vi "PCO_GetCameraDescription.vi"(8 "error in (no error)":errorcluster {"code" format="%x"}, 11 "ph":u64) -> (0 "error out":errorcluster {"code" format="%x"}, 1 "strDescription":T1 {"wSensorTypeDESC" format="%x"; "wSensorSubTypeDESC" format="%x"; "wColorPatternDESC" format="%x"; "wPatternTypeDESC" format="%x"; "dwGeneralCapsDESC1" format="%x"; "dwGeneralCapsDESC2" format="%x"; "dwGeneralCapsDESC3" format="%x"; "dwGeneralCapsDESC4" format="%x"}, 2 "ErrorMessage":i32 format="%x", 3 "ph out":u64)   [LabVIEW 2019, in "SDK.lvlib" / "CameraDescription.lvlib"]
doc: "<b>Description:</b>\nSensor and camera specific description is queried. In the returned PCO_Description structure margins for all sensor related settings and bitfields for available options of the camera are given.\n\n<b>Supported camera type:</b>\nAll cameras\n\n<b>Descriptor dependency:</b>\nNone"
uses:
  CameraDescription.lvlib
  Structures/Structures.lvlib
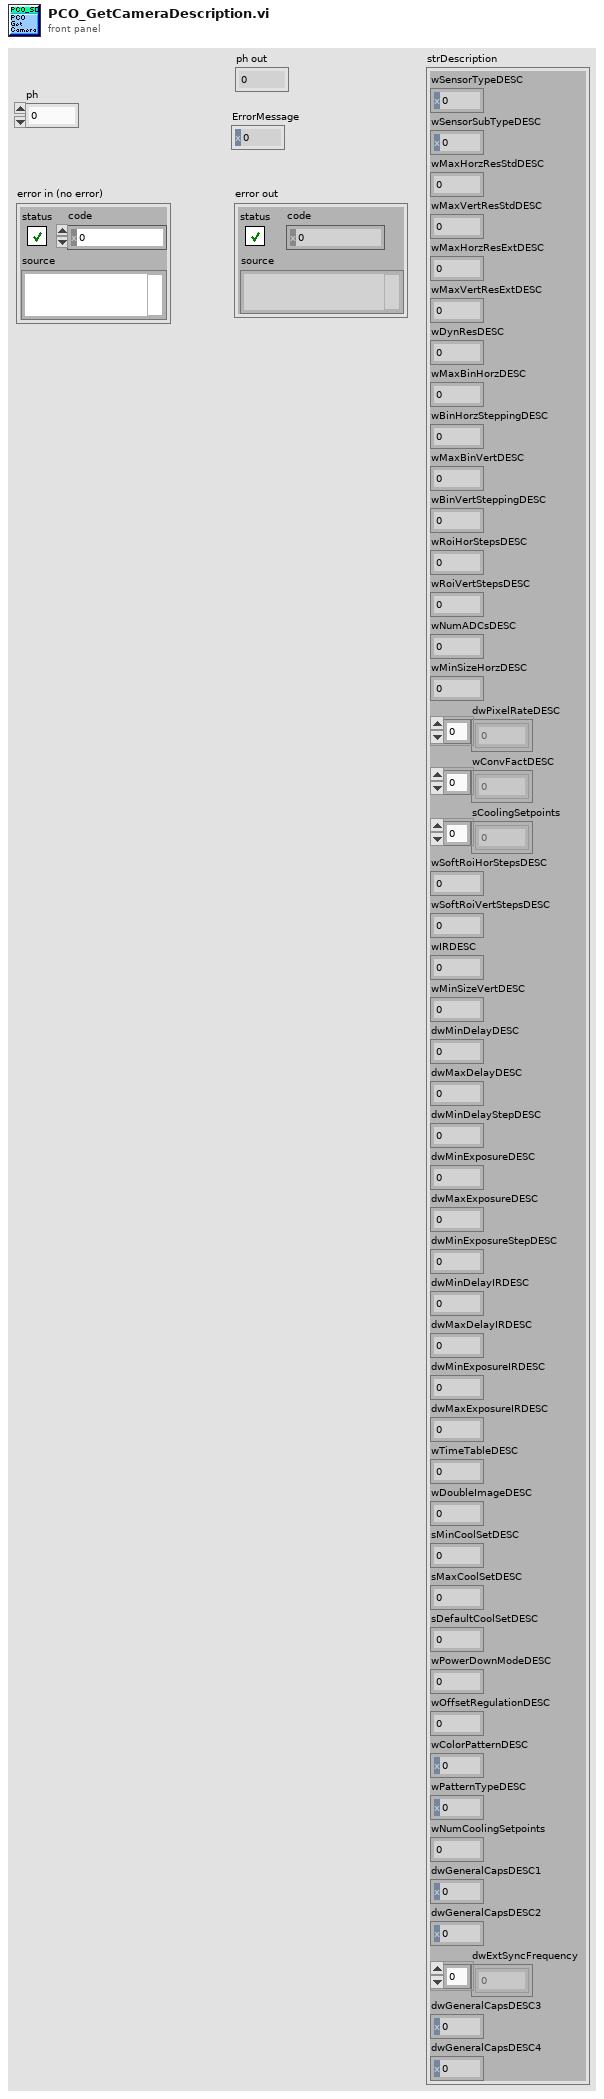
[diagram p1: front panel]
types:
  T1 = cluster{"wSensorTypeDESC":u16, "wSensorSubTypeDESC":u16, "wMaxHorzResStdDESC":u16, "wMaxVertResStdDESC":u16, "wMaxHorzResExtDESC":u16, "wMaxVertResExtDESC":u16, "wDynResDESC":u16, "wMaxBinHorzDESC":u16, "wBinHorzSteppingDESC":u16, "wMaxBinVertDESC":u16, "wBinVertSteppingDESC":u16, "wRoiHorStepsDESC":u16, "wRoiVertStepsDESC":u16, "wNumADCsDESC":u16, "wMinSizeHorzDESC":u16, "dwPixelRateDESC":u32[], "wConvFactDESC":u16[], "sCoolingSetpoints":i16[], "wSoftRoiHorStepsDESC":u16, "wSoftRoiVertStepsDESC":u16, "wIRDESC":u16, "wMinSizeVertDESC":u16, "dwMinDelayDESC":u32, "dwMaxDelayDESC":u32, "dwMinDelayStepDESC":u32, "dwMinExposureDESC":u32, "dwMaxExposureDESC":u32, "dwMinExposureStepDESC":u32, "dwMinDelayIRDESC":u32, "dwMaxDelayIRDESC":u32, "dwMinExposureIRDESC":u32, "dwMaxExposureIRDESC":u32, "wTimeTableDESC":u16, "wDoubleImageDESC":u16, "sMinCoolSetDESC":i16, "sMaxCoolSetDESC":i16, "sDefaultCoolSetDESC":i16, "wPowerDownModeDESC":u16, "wOffsetRegulationDESC":u16, "wColorPatternDESC":u16, "wPatternTypeDESC":u16, "wNumCoolingSetpoints":u16, "dwGeneralCapsDESC1":u32, "dwGeneralCapsDESC2":u32, "dwExtSyncFrequency":u32[], "dwGeneralCapsDESC3":u32, "dwGeneralCapsDESC4":u32}
  T2 = cluster{"wSize":u16, "wSensorTypeDESC":u16, "wSensorSubTypeDESC":u16, "wMaxHorzResStdDESC":u16, "wMaxVertResStdDESC":u16, "wMaxHorzResExtDESC":u16, "wMaxVertResExtDESC":u16, "wDynResDESC":u16, "wMaxBinHorzDESC":u16, "wBinHorzSteppingDESC":u16, "wMaxBinVertDESC":u16, "wBinVertSteppingDESC":u16, "wRoiHorStepsDESC":u16, "wRoiVertStepsDESC":u16, "wNumADCsDESC":u16, "wMinSizeHorzDESC":u16, "dwPixelRateDESC":cluster{u32, u32, u32, u32}, "ZZdwDummypr":cluster{u32, u32, u32, u32, u32, u32, u32, u32, u32, u32, u32, u32, u32, u32, u32, u32, u32, u32, u32, u32}, "wConvFactDESC":cluster{u16, u16, u16, u16}, "sCoolingSetpoints":cluster{i16, i16, i16, i16, i16, i16, i16, i16, i16, i16}, "ZZdwDummycv":cluster{u16, u16, u16, u16, u16, u16, u16, u16}, "wSoftRoiHorStepsDESC":u16, "wSoftRoiVertStepsDESC":u16, "wIRDESC":u16, "wMinSizeVertDESC":u16, "dwMinDelayDESC":u32, "dwMaxDelayDESC":u32, "dwMinDelayStepDESC":u32, "dwMinExposureDESC":u32, "dwMaxExposureDESC":u32, "dwMinExposureStepDESC":u32, "dwMinDelayIRDESC":u32, "dwMaxDelayIRDESC":u32, "dwMinExposureIRDESC":u32, "dwMaxExposureIRDESC":u32, "wTimeTableDESC":u16, "wDoubleImageDESC":u16, "sMinCoolSetDESC":i16, "sMaxCoolSetDESC":i16, "sDefaultCoolSetDESC":i16, "wPowerDownModeDESC":u16, "wOffsetRegulationDESC":u16, "wColorPatternDESC":u16, "wPatternTypeDESC":u16, "wDummy1":u16, "wDummy2":u16, "wNumCoolingSetpoints":u16, "dwGeneralCapsDESC1":u32, "dwGeneralCapsDESC2":u32, "dwExtSyncFrequency":cluster{u32, u32, u32, u32}, "dwGeneralCapsDESC3":u32, "dwGeneralCapsDESC4":u32, "ZZdwDummy":cluster{u32, u32, u32, u32, u32, u32, u32, u32, u32, u32, u32, u32, u32, u32, u32, u32, u32, u32, u32, u32, u32, u32, u32, u32, u32, u32, u32, u32, u32, u32, u32, u32, u32, u32, u32, u32, u32, u32, u32, u32}}
  T3 = cluster{i16, i16, i16, i16, i16, i16, i16, i16, i16, i16}
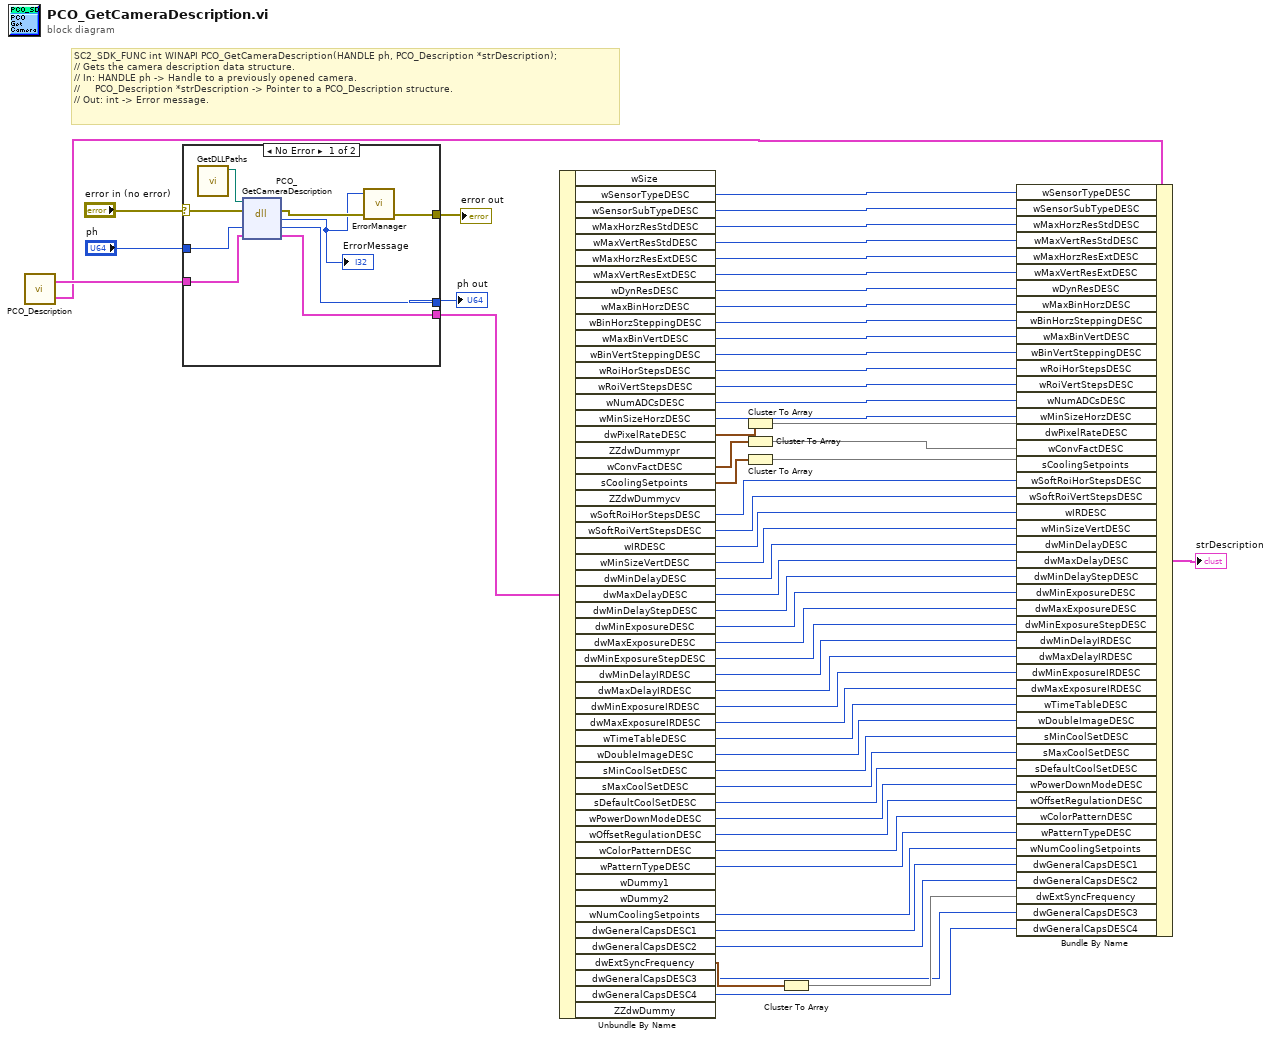
[diagram p0: block diagram]
diagram:
  # "SC2_SDK_FUNC int WINAPI PCO_GetCameraDescription(HANDLE ph, PCO_Description *strDescription);\n// Gets the camera description data structure.\n// In: HANDLE ph -> Handle to a previously opened camera.\n//     PCO_Description *strDescription -> Pointer to a PCO_Description structure.\n// Out: int -> Error message."
  n1 = call "PCO_Description.vi"() -> ("PCO_Description"=w53:T1, "PCO_Description_Raw"=w55:T2)  [unwired: 4 in, 2 out]
  n2 = case shown="No Error" "error in (no error)" {
    selector: "error in (no error)" -> [w61 w71]
    tunnel: "ph" -> [w68 w70]
    tunnel: [w67 w70] -> w58
    tunnel: w55 -> [w66 w69]
    tunnel: [w65 w69] -> w54
    tunnel: [w63 w71] -> w57
    frame No Error {
      n3 = call "GetDLLPaths.vi"() -> ("SC2_Cam_Path"=w60:path)  [unwired: 8 in, 3 out]
      n4 = dll-call lib="?" fn="PCO_GetCameraDescription"(path in=w60, error in=w61, "ph"=w68, "strDescription"=w66) -> (error out=w64:errorcluster, "return type"=w62:i32, "ph"=w67:u64, "strDescription"=w65:T2)  [unwired: 1 in, 1 out]
      "ErrorMessage" <- w62
      n5 = call "ErrorManager.vi"("error in (no error)"=w64, "error code"=w62) -> ("error out"=w63:errorcluster)  [unwired: 2 in, 1 out]
    }
    frame Error {
    }
  }
  "ph out" <- w58
  "error out" <- w57
  n6 = Unbundle By Name(w54) -> ("wSensorTypeDESC"=w51:u16, "wSensorSubTypeDESC"=w50:u16, "wMaxHorzResStdDESC"=w49:u16, "wMaxVertResStdDESC"=w48:u16, "wMaxHorzResExtDESC"=w47:u16, "wMaxVertResExtDESC"=w46:u16, "wDynResDESC"=w45:u16, "wMaxBinHorzDESC"=w44:u16, "wBinHorzSteppingDESC"=w43:u16, "wMaxBinVertDESC"=w42:u16, "wBinVertSteppingDESC"=w41:u16, "wRoiHorStepsDESC"=w40:u16, "wRoiVertStepsDESC"=w39:u16, "wNumADCsDESC"=w38:u16, "wMinSizeHorzDESC"=w37:u16, "dwPixelRateDESC"=w36:cluster{u32, u32, u32, u32}, "wConvFactDESC"=w34:cluster{u16, u16, u16, u16}, "sCoolingSetpoints"=w32:T3, "wSoftRoiHorStepsDESC"=w30:u16, "wSoftRoiVertStepsDESC"=w29:u16, "wIRDESC"=w28:u16, "wMinSizeVertDESC"=w27:u16, "dwMinDelayDESC"=w26:u32, "dwMaxDelayDESC"=w25:u32, "dwMinDelayStepDESC"=w24:u32, "dwMinExposureDESC"=w23:u32, "dwMaxExposureDESC"=w22:u32, "dwMinExposureStepDESC"=w21:u32, "dwMinDelayIRDESC"=w20:u32, "dwMaxDelayIRDESC"=w19:u32, "dwMinExposureIRDESC"=w18:u32, "dwMaxExposureIRDESC"=w17:u32, "wTimeTableDESC"=w16:u16, "wDoubleImageDESC"=w15:u16, "sMinCoolSetDESC"=w14:i16, "sMaxCoolSetDESC"=w13:i16, "sDefaultCoolSetDESC"=w12:i16, "wPowerDownModeDESC"=w11:u16, "wOffsetRegulationDESC"=w10:u16, "wColorPatternDESC"=w9:u16, "wPatternTypeDESC"=w8:u16, "wNumCoolingSetpoints"=w7:u16, "dwGeneralCapsDESC1"=w6:u32, "dwGeneralCapsDESC2"=w5:u32, "dwExtSyncFrequency"=w4:cluster{u32, u32, u32, u32}, "dwGeneralCapsDESC3"=w2:u32, "dwGeneralCapsDESC4"=w1:u32)  [unwired: 6 out]
  n7 = Cluster To Array(cluster=w36) -> (array=w35:u32[])
  n8 = Cluster To Array(cluster=w34) -> (array=w33:u16[])
  n9 = Cluster To Array(cluster=w32) -> (array=w31:i16[])
  n10 = Cluster To Array(cluster=w4) -> (array=w3:u32[])
  n11 = Bundle By Name(cluster=w53, "wSensorTypeDESC"=w51, "wSensorSubTypeDESC"=w50, "wMaxHorzResStdDESC"=w49, "wMaxVertResStdDESC"=w48, "wMaxHorzResExtDESC"=w47, "wMaxVertResExtDESC"=w46, "wDynResDESC"=w45, "wMaxBinHorzDESC"=w44, "wBinHorzSteppingDESC"=w43, "wMaxBinVertDESC"=w42, "wBinVertSteppingDESC"=w41, "wRoiHorStepsDESC"=w40, "wRoiVertStepsDESC"=w39, "wNumADCsDESC"=w38, "wMinSizeHorzDESC"=w37, "dwPixelRateDESC"=w35, "wConvFactDESC"=w33, "sCoolingSetpoints"=w31, "wSoftRoiHorStepsDESC"=w30, "wSoftRoiVertStepsDESC"=w29, "wIRDESC"=w28, "wMinSizeVertDESC"=w27, "dwMinDelayDESC"=w26, "dwMaxDelayDESC"=w25, "dwMinDelayStepDESC"=w24, "dwMinExposureDESC"=w23, "dwMaxExposureDESC"=w22, "dwMinExposureStepDESC"=w21, "dwMinDelayIRDESC"=w20, "dwMaxDelayIRDESC"=w19, "dwMinExposureIRDESC"=w18, "dwMaxExposureIRDESC"=w17, "wTimeTableDESC"=w16, "wDoubleImageDESC"=w15, "sMinCoolSetDESC"=w14, "sMaxCoolSetDESC"=w13, "sDefaultCoolSetDESC"=w12, "wPowerDownModeDESC"=w11, "wOffsetRegulationDESC"=w10, "wColorPatternDESC"=w9, "wPatternTypeDESC"=w8, "wNumCoolingSetpoints"=w7, "dwGeneralCapsDESC1"=w6, "dwGeneralCapsDESC2"=w5, "dwExtSyncFrequency"=w3, "dwGeneralCapsDESC3"=w2, "dwGeneralCapsDESC4"=w1) -> (→"strDescription":T1)
